vi "CreateUserEvents.vi"(8 "error in (no error)":errorcluster, 11 "UserEvents":T1) -> (0 "error out":errorcluster, 3 "UserEvents out":T1)   [LabVIEW 2022 SP3, in "TopLevel.lvclass"]
uses:
  TopLevel.lvclass
  Typedefs/UserEvents.ctl
  Typedefs/API Event Data.ctl
  Typedefs/API Task State.ctl
  Motor Controller/Typedefs/Status_TopLevel--Cluster.ctl
  Common/Controls/TD MasterConfiguration DLPC2--cluster.ctl
  Common/Controls/DLPC2_Path--Cluster.ctl
  Common/Controls/TD HeadColorPaneMappingAll--cluster.ctl
  Common/Controls/TD HeadColorPaneMapping--cluster.ctl
  Typedefs/SpitVoltages--Cluster.ctl
  Typedefs/PrimingMode APIData.ctl
  Typedefs/PurgeMode--Enum.ctl
  Typedefs/PrinterHeads--Enum.ctl
  Common/Controls/GenericEventData--Cluster.ctl
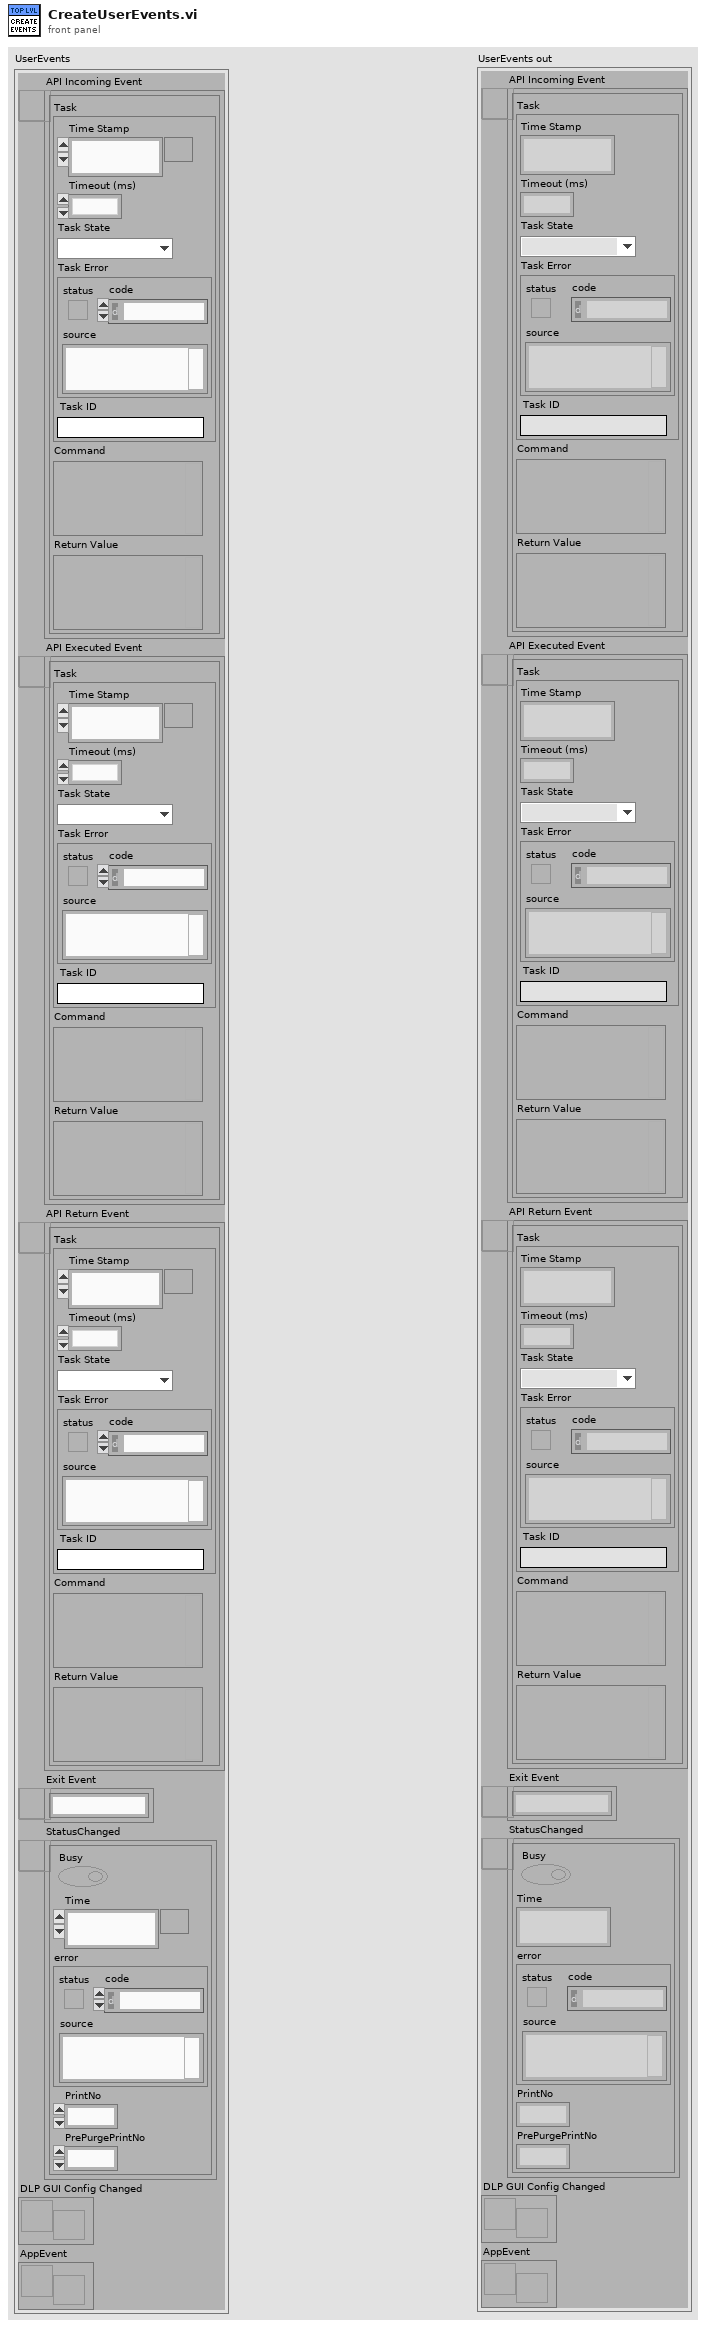
[diagram p1: front panel]
types:
  T1 = typedef "TopLevel.lvclass/UserEvents.ctl" = cluster{"API Incoming Event":refnum<user-event>, "API Executed Event":refnum<user-event>, "API Return Event":refnum<user-event>, "Exit Event":refnum<user-event>, "StatusChanged":refnum<user-event>, "DLP GUI Config Changed":refnum<user-event>, "AppEvent":refnum<user-event>}
  T2 = typedef "Status_TopLevel--Cluster.ctl" = cluster{"Busy":bool, "Time":timestamp, "error":errorcluster, "PrintNo":i32, "PrePurgePrintNo":i32}
  T3 = typedef "TopLevel.lvclass/API Event Data.ctl" = cluster{"Task":cluster{"Time Stamp":timestamp, "Timeout (ms)":u32, "Task State":T4, "Task Error":errorcluster, "Task ID":string}, "Command":variant, "Return Value":variant}
  T4 = typedef "TopLevel.lvclass/API Task State.ctl" = enum16{"Completed", "Errored", "Pending"}
  T5 = typedef "GenericEventData--Cluster.ctl" = cluster{"Command":string, "Data":variant}
  T6 = typedef "TD MasterConfiguration DLPC2--cluster.ctl" = cluster{"Paths":T7, "ColorPaneMapping":T8, "Materials":string[], "ColorPlanes":string[], "SpitVoltages_Half":T10, "SpitVoltages_Full":T10, "SystemMode":string[], "PrimeModeConfig":T11[], "Running Average Duration_s":dbl}
  T7 = typedef "DLPC2_Path--Cluster.ctl" = cluster{"DigiBit WG Design Folder":path, "Compensated GS Image Folder":path, "Nozzle GS Files Head 1":path, "Nozzle GS Files Head 2":path, "Nozzle GS Files Head 3":path, "Nozzle GS Files Head 4":path, "Nozzle GS Files Head 5":path, "Nozzle GS Files Head 6":path}
  T8 = typedef "TD HeadColorPaneMappingAll--cluster.ctl" = cluster{"Head 1":T9, "Head 2":T9, "Head 3":T9, "Head 4":T9, "Head 5":T9, "Head 6":T9}
  T9 = typedef "TD HeadColorPaneMapping--cluster.ctl" = cluster{"Material":string, "ColorPane":string}
  T10 = typedef "SpitVoltages--Cluster.ctl" = cluster{"1":dbl, "2":dbl, "3":dbl, "4":dbl, "5":dbl, "6":dbl}
  T11 = typedef "TopLevel.lvclass/PrimingMode APIData.ctl" = cluster{"Interval (s)":dbl, "PurgeDuration (s)":dbl, "Repeats":u8, "PrimingMode":T12, "Head":T13}
  T12 = typedef "PurgeMode--Enum.ctl" = enum16{"Pre-Purge", "Purge", "Spit", "Prime"}
  T13 = typedef "PrinterHeads--Enum.ctl" = enum16{"-1", "1", "2", "3", "4", "5", "6"}
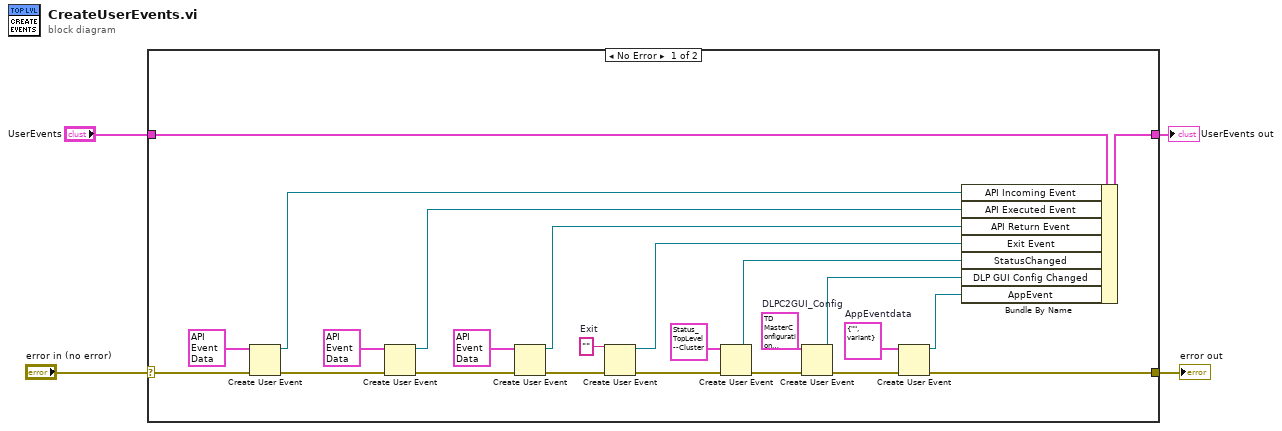
[diagram p0: block diagram]
diagram:
  n1 = case shown="No Error" "error in (no error)" {
    selector: "error in (no error)" -> [w24 w30]
    tunnel: [w6 w30] -> w3
    tunnel: "UserEvents" -> [w28 w29]
    tunnel: [w27 w29] -> w1
    frame No Error {
      w8 = T5 {"Command"="", "Data"=variant}  # AppEventdata
      w10 = T6 {"Paths"={"DigiBit WG Design Folder"=path "C:/projects/Digilens_IPLC", "Compensated GS Image Folder"=path "C:/projects/Digilens_IPLC", "Nozzle GS Files Head 1"=path "C:/projects/Digilens_IPLC/DLPC2Config.xml", "Nozzle GS Files Head 2"=path "C:/projects/Digilens_IPLC/DLPC2Config.xml", "Nozzle GS Files Head 3"=path "C:/projects/Digilens_IPLC/DLPC2Config.xml", "Nozzle GS Files Head 4"=path "C:/projects/Digilens_IPLC/DLPC2Config.xml", "Nozzle GS Files Head 5"=path "C:/projects/Digilens_IPLC/DLPC2Config.xml", "Nozzle GS Files Head 6"=path "C:/projects/Digilens_IPLC/DLPC2Config.xml"}, "ColorPaneMapping"={"Head 1"={"Material"="109G", "ColorPane"="0-C"}, "Head 2"={"Material"="311A", "ColorPane"="1-M"}, "Head 3"={"Material"="FD/OP-3", "ColorPane"="2-Y"}, "Head 4"={"Material"="311A", "ColorPane"="3-K"}, "Head 5"={"Material"="507 - 100%", "ColorPane"="4-Blue-Spot"}, "Head 6"={"Material"="507 - 50%", "ColorPane"="5-Orange-Spot"}}, "Materials"=[], "ColorPlanes"=[], "SpitVoltages_Half"={"1"=0.0, "2"=0.0, "3"=0.0, "4"=0.0, "5"=0.0, "6"=0.0}, "SpitVoltages_Full"={"1"=0.0, "2"=0.0, "3"=0.0, "4"=0.0, "5"=0.0, "6"=0.0}, "SystemMode"=[], "PrimeModeConfig"=[], "Running Average Duration_s"=5.0}  # DLPC2GUI_Config
      w17 = ""  # Exit
      n2 = Create User Event(user event datatype=T3 {"Task"={"Time Stamp"=timestamp(0 s since 1904-01-01), "Timeout (ms)"=0, "Task State"=enum."Completed", "Task Error"={"status"=FALSE, "code"=0, "source"=""}, "Task ID"=""}, "Command"=variant(enum16{"Event 1"} enum."Event 1"), "Return Value"=variant(string "")} ("API Event Data"), error in=w24) -> (user event=w25:refnum<user-event>, error out=w22:errorcluster)
      n3 = Create User Event(user event datatype=T3 {"Task"={"Time Stamp"=timestamp(0 s since 1904-01-01), "Timeout (ms)"=0, "Task State"=enum."Completed", "Task Error"={"status"=FALSE, "code"=0, "source"=""}, "Task ID"=""}, "Command"=variant(enum16{"Event 1"} enum."Event 1"), "Return Value"=variant(string "")} ("API Event Data"), error in=w22) -> (user event=w21:refnum<user-event>, error out=w19:errorcluster)
      n4 = Create User Event(user event datatype=T3 {"Task"={"Time Stamp"=timestamp(0 s since 1904-01-01), "Timeout (ms)"=0, "Task State"=enum."Completed", "Task Error"={"status"=FALSE, "code"=0, "source"=""}, "Task ID"=""}, "Command"=variant(enum16{"Event 1"} enum."Event 1"), "Return Value"=variant(string "")} ("API Event Data"), error in=w19) -> (user event=w18:refnum<user-event>, error out=w16:errorcluster)
      n5 = Create User Event(user event datatype=w17, error in=w16) -> (user event=w15:refnum<user-event>, error out=w13:errorcluster)
      n6 = Create User Event(user event datatype=T2 {"Busy"=FALSE, "Time"=timestamp(0 s since 1904-01-01), "error"={"status"=FALSE, "code"=0, "source"=""}, "PrintNo"=0, "PrePurgePrintNo"=0} ("Status"), error in=w13) -> (user event=w12:refnum<user-event>, error out=w11:errorcluster)
      n7 = Create User Event(user event datatype=w10, error in=w11) -> (user event=w9:refnum<user-event>, error out=w7:errorcluster)
      n8 = Create User Event(user event datatype=w8, error in=w7) -> (user event=w5:refnum<user-event>, error out=w6:errorcluster)
      n9 = Bundle By Name(cluster=w28, "API Incoming Event"=w25, "API Executed Event"=w21, "API Return Event"=w18, "Exit Event"=w15, "StatusChanged"=w12, "DLP GUI Config Changed"=w9, "AppEvent"=w5) -> (w27:T1)
    }
    frame Error {
    }
  }
  "error out" <- w3
  "UserEvents out" <- w1
